vi "onProcessStarted.vi"(8 "error in (no error)":errorcluster, 11 "MAUI":refnum<class "MAUI.lvclass">) -> (0 "error out":errorcluster, 3 "MAUI out":refnum<class "MAUI.lvclass">)   [LabVIEW 2016, in "MAUI.lvclass"]
doc: "JKI State Machine Objects (SMO) 1.3.0.56\nJKI - JKI\nCopyright (c) 2017, JKI"
uses:
  MAUI.lvclass
  <vilib>/JKI/JKI SMO/SMO.UI/SMO.UI.lvclass
  <vilib>/Levylab/Embedded SMO UI/EmbeddedSMO.lvclass
  <vilib>/JKI/JKI SMO/SMO/SMO.lvclass
  C:/Program Files (x86)/National Instruments/LabVIEW 2016/vi.lib/JKI/JKI SMO/SMO/SMO.lvclass
panel:
  # "For instructions on how to use the JKI State Machine Objects, examples and video tutorials, visit:\nhttp://jki.net/state-machine-objects/\n\nJKI State Machine Objects™\nhttp://jki.net/state-machine-objects/\nCopyright (C) 2005-2015, JKI <info@jki.net>\nALL RIGHTS RESERVED"
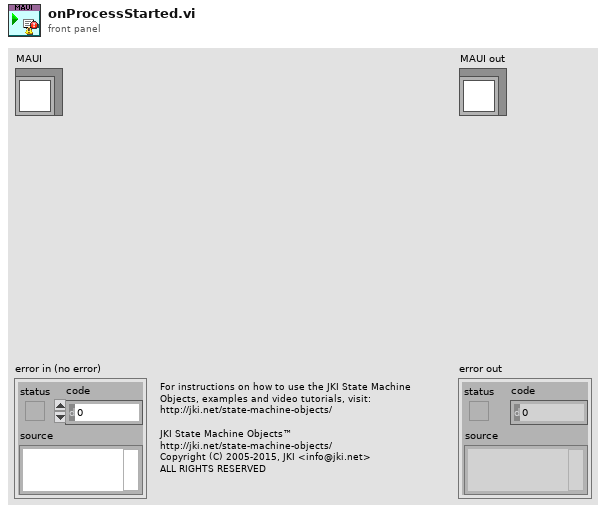
[diagram p1: front panel]
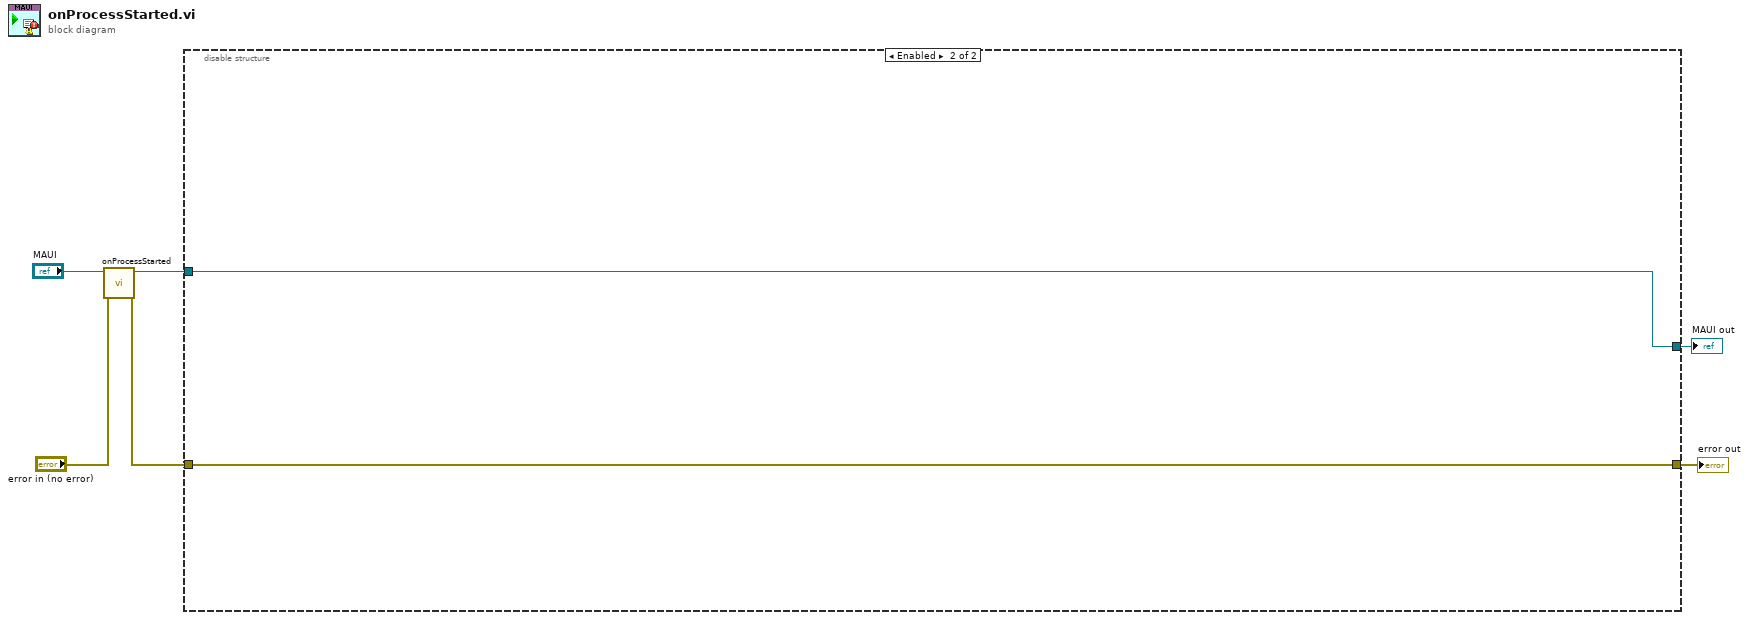
[diagram p0: block diagram]
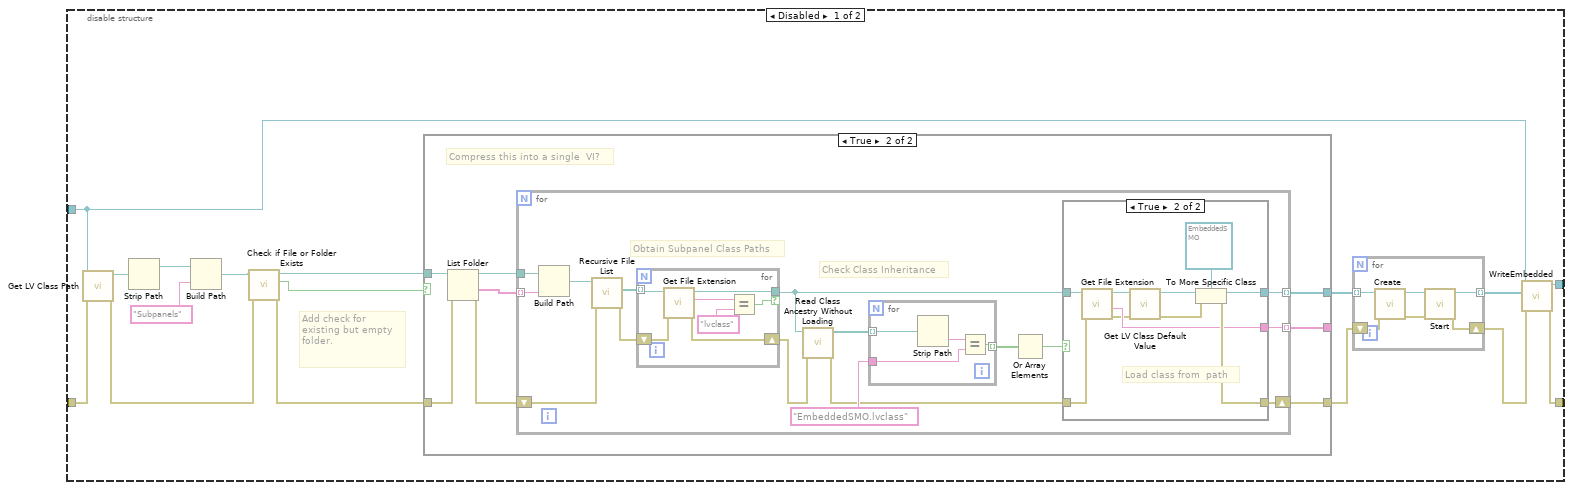
[diagram p2: hidden frame]
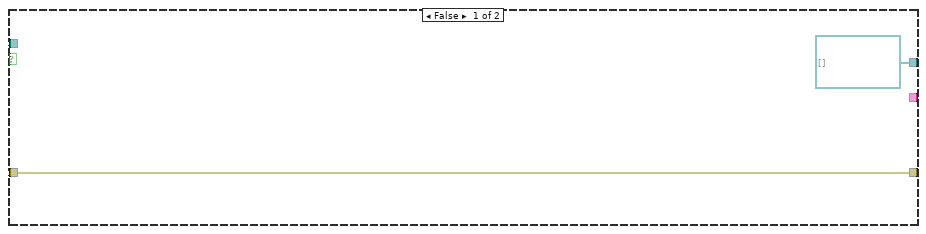
[diagram p3: hidden frame]
diagram:
  n1 = call-parent "onProcessStarted.vi"("error in (no error)"="error in (no error)", "SMO"="MAUI") -> ("error out"=w4:errorcluster, "SMO out"=w3:refnum<class "MAUI.lvclass">)  [unwired: 8 in]
  n2 = disable-structure shown="Enabled" {
    disable-tunnel: w4 -> [w14 w78]
    disable-tunnel: w3 -> [w13 w79]
    disable-tunnel: [w12 w78] -> w2
    disable-tunnel: [w11 w79] -> w1
    frame Disabled {
      # "Add check for existing but empty folder."
      n3 = call <vilib>:"Get LV Class Path.vi"("error in (no error)"=w14, "object"=w13) -> ("error out"=w15:errorcluster, "class path"=w22:path)  [unwired: 8 in]
      n4 = Strip Path(path=w22) -> (stripped path=w21:path)  [unwired: 1 out]
      n5 = Build Path(base path=w21, name or relative path="Subpanels") -> (appended path=w19:path)
      n6 = call <vilib>:"Check if File or Folder Exists.vi"("error in (no error)"=w15, "path"=w19) -> ("error out"=w17:errorcluster, "file or folder exists?"=w16:bool, "dup path"=w18:path)  [unwired: 7 in]
      n7 = case shown="True" w16 {
        tunnel: w18 -> [w31 w39]
        tunnel: w17 -> [w30 w34]
        tunnel: [w30 w33] -> w7
        tunnel: [refnum<class "EmbeddedSMO.lvclass">[] [] w35] -> w10
        tunnel: [_ w32] -> _
        frame False {
          n8 = Create Folder(path (use dialog)=w31, error in=w30) -> ()  [unwired: 1 in, 3 out]
        }
        frame True {
          # "Compress this into a single  VI?"
          n9 = List Folder(path=w39, error in=w34) -> (path out=w38:path, folder names=w37:string[], error out=w36:errorcluster)  [unwired: 2 in, 1 out]
          n10 = for {
            tunnel: w38 -> [w55]
            tunnel: w37 -> [w54] mode=indexing
            tunnel: [w50] -> w35 mode=indexing
            shift-right: [w42] -> w33
            shift-left: w36 -> [w46]
            tunnel: [w40] -> w32 mode=indexing
            # "Check Class Inheritance"
            # "Obtain Subpanel Class Paths"
            n11 = Build Path(base path=w55, name or relative path=w54) -> (appended path=w53:path)
            n12 = call <vilib>:"Recursive File List.vi"("error in (no error)"=w46, "Folder Path"=w53) -> ("error out"=w45:errorcluster, "All Files in Dir"=w52:path[])  [unwired: 5 in, 3 out]
            n13 = for {
              tunnel: w52 -> [w75] mode=indexing
              tunnel: [w74] -> w51 if=w73
              shift-right: [w71] -> w44
              shift-left: w45 -> [w72]
              n14 = call <vilib>:"Get File Extension.vi"("error in (no error)"=w72, "file"=w75) -> ("error out"=w71:errorcluster, "lowercase file extension"=w77:string, "dup file"=w74:path)  [unwired: 5 in, 2 out]
              n15 = Equal?(x=w77, y="lvclass") -> (x = y?=w73:bool)
            }
            n16 = call <vilib>:"Read Class Ancestry Without Loading.vi"("error in (no error)"=w44, "LabVIEW Class Path"=w51) -> ("error out"=w43:errorcluster, "Class Ancestry"=w49:path[])  [unwired: 8 in]
            n17 = for {
              tunnel: w49 -> [w70] mode=indexing
              tunnel: [w68] -> w48 mode=indexing
              tunnel: "EmbeddedSMO.lvclass" -> [w67]
              n18 = Strip Path(path=w70) -> (name=w69:string)  [unwired: 1 out]
              n19 = Equal?(x=w69, y=w67) -> (x = y?=w68:bool)
            }
            n20 = Or Array Elements(Boolean array=w48) -> (logical OR=w41:bool)
            n21 = case shown="True" w41 {
              tunnel: w51 -> [_ w61]
              tunnel: [_ w66] -> w50
              tunnel: w43 -> [w56 w58]
              tunnel: [w56 w62] -> w42
              tunnel: [_ w59] -> w40
              frame False {
              }
              frame True {
                # "Load class from  path"
                n22 = call <vilib>:"Get File Extension.vi"("error in (no error)"=w58, "file"=w61) -> ("error out"=w57:errorcluster, "filename without extension"=w59:string, "dup file"=w60:path)  [unwired: 5 in, 2 out]
                n23 = call <vilib>:"Get LV Class Default Value.vi"("error in (no error)"=w57, "class path"=w60) -> ("error out"=w63:errorcluster, "object"=w65:refnum<class>)  [unwired: 8 in]
                n24 = To More Specific Class(target class=refnum<class "EmbeddedSMO.lvclass"> refnum ("EmbeddedSMO"), reference=w65, error in=w63) -> (specific class reference=w66:refnum<class "EmbeddedSMO.lvclass">, error out=w62:errorcluster)
              }
            }
          }
        }
      }
      n25 = for {
        tunnel: w10 -> [w28] mode=indexing
        tunnel: [w27] -> w9 mode=indexing
        shift-right: [w23] -> w8
        shift-left: w7 -> [w24]
        n26 = call <vilib>:"Create.vi"("error in (no error)"=w24, "SMO"=w28) -> ("error out"=w25:errorcluster, "SMO out"=w26:refnum<class "EmbeddedSMO.lvclass">)  [unwired: 7 in, 1 out]
        n27 = call <vilib>:"Start.vi"("error in (no error)"=w25, "SMO"=w26) -> ("error out"=w23:errorcluster, "SMO out"=w27:refnum<class "EmbeddedSMO.lvclass">)  [unwired: 8 in]
      }
      n28 = call "WriteEmbedded.vi"("error in (no error)"=w8, "Subpanels"=w9, "MAUI in"=w13) -> ("error out"=w12:errorcluster, "MAUI out"=w11:refnum<class "MAUI.lvclass">)  [unwired: 7 in]
    }
    frame Enabled {
    }
  }
  "error out" <- w2
  "MAUI out" <- w1
